vi "Enqueue Array.vi"(8 "error in":errorcluster, 9 "Messages Data":variant[](array[variant]), 10 "Messages":string[](array[string]), 11 "Priority?":bool[](array[boolean])) -> (0 "error out":errorcluster)   [LabVIEW 2020, in "MHL.lvlib"]
doc: "Enqueue an array of states for the FGV queue based state machine.\n\n\n--------------------\nJuan Navarro\nLab It Studio"
uses:
  MHL.lvlib
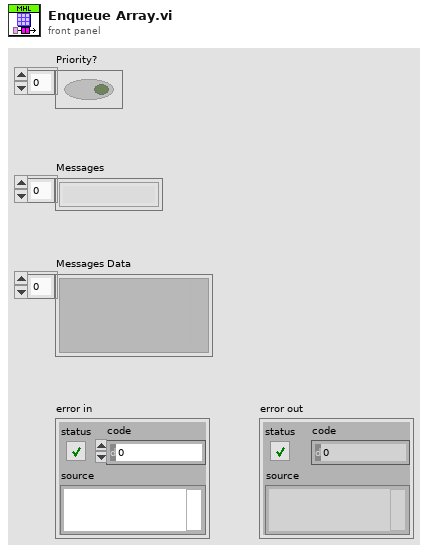
[diagram p1: front panel]
types:
  T1 = enum16{"Obtain", "Enqueue", "Get Queue", "Flush", "Release"}
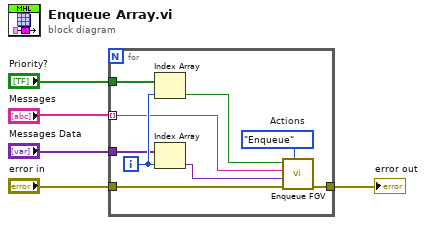
[diagram p0: block diagram]
diagram:
  n1 = for {
    tunnel: "Messages" -> [w7] mode=indexing
    tunnel: [w14] -> w2
    tunnel: "error in" -> [w13]
    tunnel: "Messages Data" -> [w10]
    tunnel: "Priority?" -> [w12]
    i -> [w11]
    w6 = T1."Enqueue"  # Actions
    n2 = Index Array(array=w12, index=w11) -> (element=w9:bool)
    n3 = Index Array(array=w10, index=w11) -> (element=w8:variant)
    n4 = call "Enqueue FGV.vi"("Actions"=w6, "error in"=w13, "Message Data"=w8, "Message"=w7, "Priority?"=w9) -> ("error out"=w14:errorcluster)  [unwired: 5 in, 1 out]
  }
  "error out" <- w2
